vi "SingleWithPayload.vi"() -> (1 "ActionStack out":refnum<class "Stack.lvclass">)   [LabVIEW 2025]
uses:
  Stack.lvclass/Stack.ctl
  Stack.lvclass
  Action/Action.lvclass
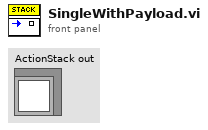
[diagram p1: front panel]
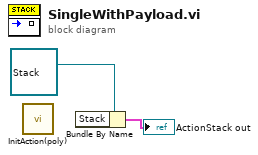
[diagram p0: block diagram]
diagram:
  n1 = call-poly "InitAction(poly).vi"() -> ()  [unwired: 11 in, 1 out]
  n2 = Bundle By Name(cluster=refnum<class "Stack.lvclass"> refnum ("ActionStack.lvclass")) -> (→"ActionStack out":cluster{})  [unwired: 1 in]
